vi "GUNSC_LibAddDet.vi"(0 "detector":T1, 5 "Amplifier":T2={"number"=0, "type"=0, "rotated"=0, "fliped"=0, "FPAcoord"={"xstart"=1, "ystart"=1}, "Physical_size"={"columns"=0, "rows"=0}, "predata"={"columns"=0, "rows"=0}, "postdata"={"columns"=0, "rows"=0}, "Req ROIs"=[], "Corr ROI"=[], "Detnumber"=0, "ampID"="", "discard"=0} {"fliped" items=["none", "horizontal", "vertical"]; "type" items=["LL", "LR", "UL", "UR"]}, 11 "error in (no error)":errorcluster) -> (6 "return value":i32, 15 "error out":errorcluster)   [LabVIEW 2016]
uses:
  GEOM/private/vis/GEOM_Amplifier.ctl
  GEOM/private/vis/GEOM_AmpType.ctl
  GEOM/private/vis/GEOM_ROI.ctl
  GEOM/private/vis/GEOM_Coords.ctl
  GEOM/private/vis/GEOM_DetSummaryStruct.ctl
  public/c/lib/libunsc.so
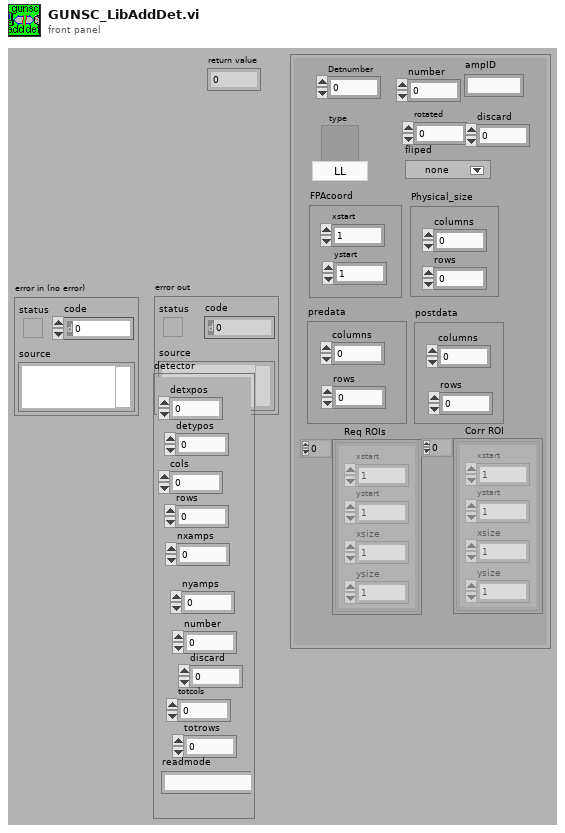
[diagram p1: front panel]
types:
  T1 = typedef "GEOM_DetSummaryStruct.ctl" = cluster{"detxpos":i32, "detypos":i32, "cols":i32, "rows":i32, "nxamps":i32, "nyamps":i32, "number":i32, "discard":i32, "totcols":i32, "totrows":i32, "readmode":string}
  T2 = typedef "GEOM_Amplifier.ctl" = cluster{"number":i32, "type":T3, "rotated":i16, "fliped":u16, "FPAcoord":cluster{"xstart":i32, "ystart":i32}, "Physical_size":cluster{"columns":i32, "rows":i32}, "predata":cluster{"columns":i32, "rows":i32}, "postdata":cluster{"columns":i32, "rows":i32}, "Req ROIs":T4, "Corr ROI":T4, "Detnumber":i32, "ampID":string, "discard":i32}
  T3 = typedef "GEOM_AmpType.ctl" = u16
  T4 = typedef "GEOM_ROI.ctl" = T5[]
  T5 = typedef "GEOM_Coords.ctl" = cluster{"xstart":u32, "ystart":u32, "xsize":u32, "ysize":u32}
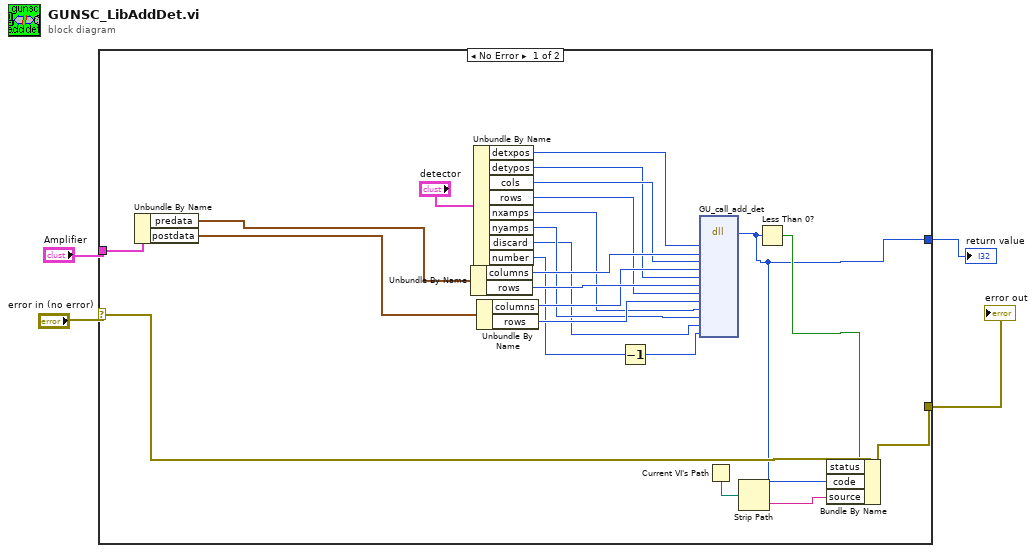
[diagram p0: block diagram]
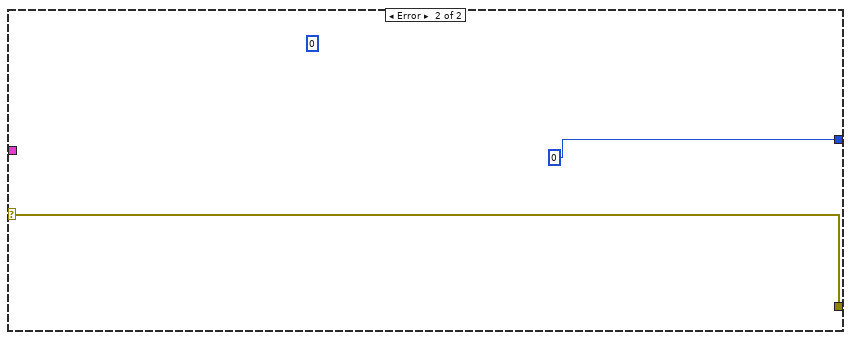
[diagram p2: hidden frame]
diagram:
  n1 = case shown="No Error" "error in (no error)" {
    selector: "error in (no error)" -> [w27 w29]
    tunnel: [w21 0] -> w4
    tunnel: [w24 w29] -> w2
    tunnel: "Amplifier" -> [w23 _]
    frame No Error {
      n2 = Unbundle By Name(w23) -> ("predata"=w18:cluster{"columns":i32, "rows":i32}, "postdata"=w15:cluster{"columns":i32, "rows":i32})
      n3 = Unbundle By Name(w18) -> ("columns"=w20:i32, "rows"=w19:i32)
      n4 = Unbundle By Name("detector") -> ("detxpos"=w13:i32, "detypos"=w11:i32, "cols"=w12:i32, "rows"=w10:i32, "nxamps"=w9:i32, "nyamps"=w8:i32, "discard"=w7:i32, "number"=w6:i32)
      n5 = Unbundle By Name(w15) -> ("columns"=w17:i32, "rows"=w16:i32)
      n6 = Decrement(x=w6) -> (x-1=w5:i32)
      n7 = dll-call lib="home/simager/panview/PAN/Modules/GUNSC/public/c/lib/libunsc.so" fn="GU_call_add_det"("xstart"=w13, "precols"=w20, "datacols"=w12, "postcols"=w17, "ystart"=w11, "prerows"=w19, "datarows"=w10, "postrows"=w16, "nxamps"=w9, "nyamps"=w8, "discard"=w7, "detno"=w5) -> ("return type"=w21:i32)  [unwired: 15 in, 2 out]
      n8 = Current VI's Path() -> (path=w26:path)
      n9 = Strip Path(path=w26) -> (name=w25:string)  [unwired: 1 out]
      n10 = Less Than 0?(x=w21) -> (x < 0?=w22:bool)
      n11 = Bundle By Name(cluster=w27, "status"=w22, "code"=w21, "source"=w25) -> (w24:errorcluster)
    }
    frame Error {
      (unwired) 0
    }
  }
  "return value" <- w4
  "error out" <- w2
